vi "simpleAuthMain.vi"(8 "Error In":errorcluster) -> (0 "Error Out":errorcluster)   [LabVIEW 2018]
panel:
  in  "Log-in Button":bool
  in  "PASSWORD :":string
  # "AUTHENTICATION"
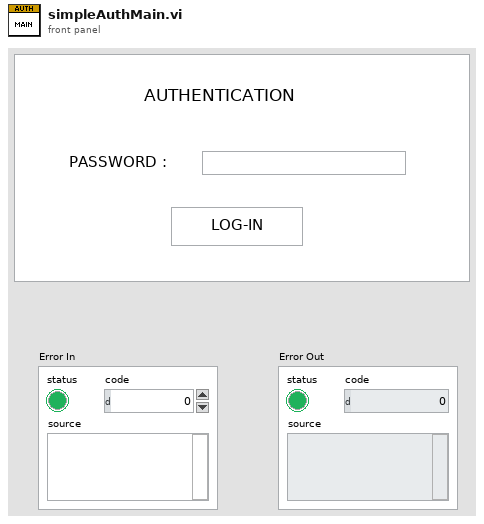
[diagram p1: front panel]
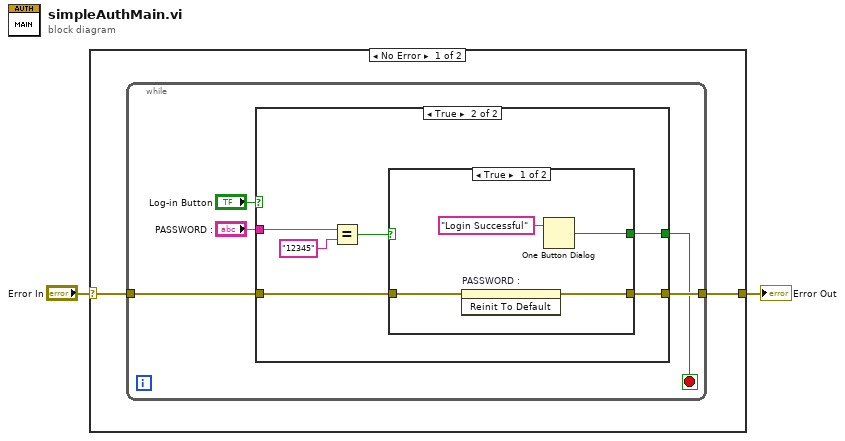
[diagram p0: block diagram]
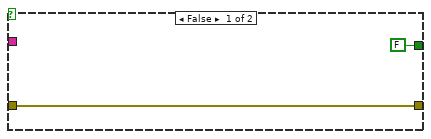
[diagram p2: hidden frame]
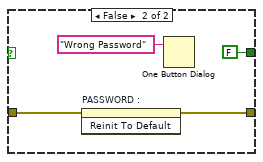
[diagram p3: hidden frame]
diagram:
  n1 = case shown="No Error" "Error In" {
    selector: "Error In" -> [w4 w26]
    tunnel: [w3 w26] -> w1
    frame No Error {
      n2 = while {
        tunnel: w4 -> [w7]
        tunnel: [w6] -> w3
        stop <- w5 stop-if-true
        n3 = case shown="True" "Log-in Button" {
          tunnel: "PASSWORD :" -> [_ w17]
          tunnel: w7 -> [w11 w13]
          tunnel: [w11 w12] -> w6
          tunnel: [FALSE ("true") w14] -> w5
          frame False {
          }
          frame True {
            n4 = Equal?(x=w17, y="12345") -> (x = y?=w15:bool)
            n5 = case shown="True" w15 {
              tunnel: [w20 FALSE ("true")] -> w14
              tunnel: w13 -> [w19 w24]
              tunnel: [w18 w23] -> w12
              frame True {
                n6 = invoke on="PASSWORD :" class="Str" method="Reinit To Default"(error in=w19) -> (error out=w18:errorcluster)  [unwired: 2 in, 2 out]
                n7 = One Button Dialog(message="Login Successful") -> (true=w20:bool)  [unwired: 1 in]
              }
              frame False {
                n8 = invoke on="PASSWORD :" class="Str" method="Reinit To Default"(error in=w24) -> (error out=w23:errorcluster)  [unwired: 2 in, 2 out]
                n9 = One Button Dialog(message="Wrong Password") -> ()  [unwired: 1 in, 1 out]
              }
            }
          }
        }
      }
    }
    frame Error {
    }
  }
  "Error Out" <- w1
